vi "Demodlator.vi"(8 "error in (no error)":errorcluster, 10 "Waveform in":waveform(dbl), 11 "ISO 15693 DOWN in":refnum<class "ISO 15693 DOWN.lvclass">) -> (0 "error out":errorcluster, 2 "Waveform out":waveform(dbl), 3 "ISO 15693 DOWN out":refnum<class "ISO 15693 DOWN.lvclass">)   [LabVIEW 2019, in "ISO 15693 DOWN.lvclass"]
uses:
  ISO 15693 DOWN.lvclass
  TypeDef/Store.ctl
  ISO 15693 DOWN.lvclass/ISO 15693 DOWN.ctl
  <vilib>/addons/Modulation/Analog/support/mod_Set Error Source.vi
  <vilib>/addons/Modulation/Analog/MT Downconvert Passband (Real).vi
  <vilib>/addons/Modulation/Analog/MT Demodulate AM (DSB).vi
  <vilib>/addons/Modulation/Digital/Support/Common/Validators/mod_Generate Filter Coefficients Validate.vi
  <vilib>/addons/Modulation/Digital/General/subVIs/mod_Generate Filter Coefficients.vi
  <vilib>/addons/Modulation/Digital/General/MT Generate ASK system parameters (M).vi
  <vilib>/addons/Modulation/niAMT.lvlib
  <vilib>/addons/Modulation/niDMT.lvlib
  RFID system.lvclass
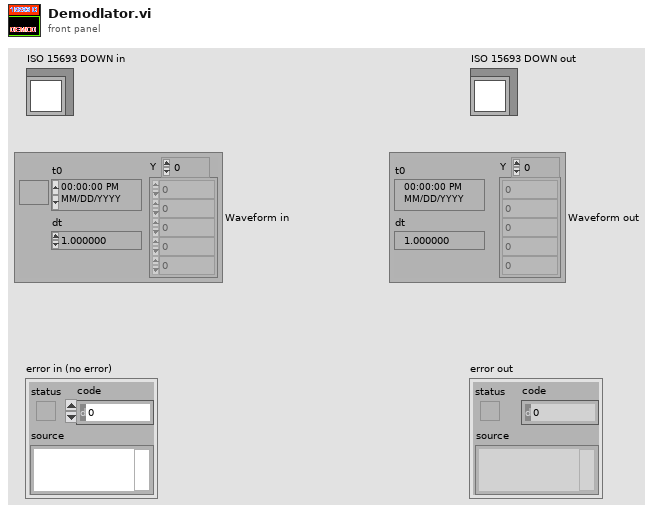
[diagram p1: front panel]
types:
  T1 = typedef "Store.ctl" = enum16{"envelope", "noise", "demSubCar", "CH_frame", "Decode", "demodulate", "in", "out", "sum", "subCarrier", "frame", "command", "encode", "modulate", "encode_UP", "modulate_up", "demod_up", "envelop_up", "sum_up", "out_up", "in_up"}
  T2 = enum16{"none", "Raised Cosine", "Root Raised Cos", "Gaussian"}
  T3 = enum16{"FSK", "PSK", "QAM", "MSK", "PAM", "ASK", "CPM"}
  T4 = cluster{"passband ripple (dB)":dbl, "stopband start (Hz)":dbl, "stopband gain (dB)":dbl, "compute filter stopband ? (T)":bool}
  T5 = typedef "niAMT.lvlib/Complex Data Waveform.ctl" = cluster{"t0":dbl, "dt":dbl, "Y":cdb[]}
  T6 = cluster{"samples per symbol (16)":i32, "symbol map":cdb[]}
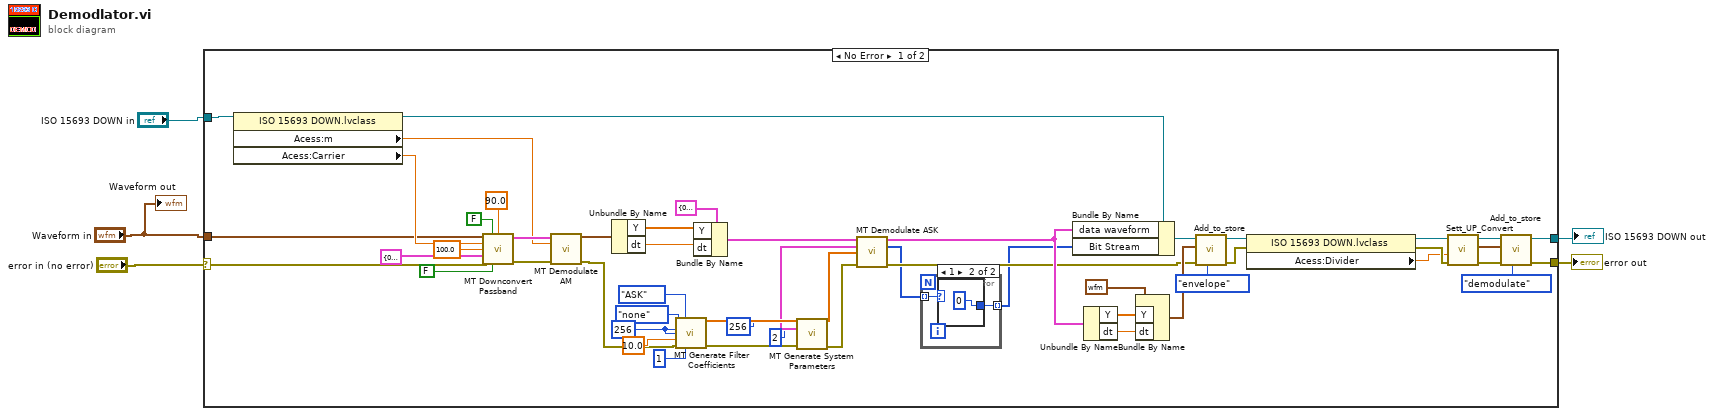
[diagram p0: block diagram]
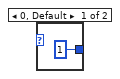
[diagram p2: hidden frame]
diagram:
  n1 = case shown="No Error" "error in (no error)" {
    selector: "error in (no error)" -> [w10 w61]
    tunnel: "ISO 15693 DOWN in" -> [w12 w62]
    tunnel: [w9 w62] -> w2
    tunnel: "Waveform in" -> [w11 _]
    tunnel: [w8 w61] -> w3
    frame No Error {
      w40 = 256 ("pulse shaping samples per symbol (16)")
      n2 = property class="ISO 15693 DOWN.lvclass"(reference=w12) -> (reference out=w32:refnum<class "ISO 15693 DOWN.lvclass">, "Acess:m"=w14:dbl, "Acess:Carrier"=w13:dbl)  [unwired: 1 in, 1 out]
      n3 = call-poly <vilib>:"MT Downconvert Passband.vi"("Waveform"=w11, "reset? (F)"=FALSE, "initial phase (deg)"=90.0, "carrier frequency (Hz)"=w13, "passband bandwidth (Hz)"=100.0, "advanced filter parameters"=T4 {"passband ripple (dB)"=0.01, "stopband start (Hz)"=0.0, "stopband gain (dB)"=-96.0, "compute filter stopband ? (T)"=TRUE}, "error in (no error)"=w10, "enable filter (T)"=FALSE) -> ("downconverted waveform (complex baseband)"=w56:T5, "error out"=w55:errorcluster)  [unwired: 4 in, 2 out]
      n4 = call-poly <vilib>:"MT Demodulate AM.vi"("AM modulated waveform"=w56, "modulation index"=w14, "error in (no error)"=w55) -> ("AM demodulated waveform"=w35:waveform(dbl), "error out"=w34:errorcluster)  [unwired: 10 in, 1 out]
      n5 = Unbundle By Name(w35) -> ("Y"=w47:dbl[], "dt"=w48:dbl)
      n6 = call <vilib>:"MT Generate Filter Coefficients.vi"("pulse shaping filter (none)"=T2."none", "modulation type"=T3."ASK", "pulse shaping samples per symbol (16)"=w40, "matched samples per symbol (16)"=w40, "filter parameter"=10.0, "error in (no error)"=w34, "filter length (symbols)"=1) -> ("pulse shaping filter coefficients"=w46:dbl[], "error out"=w44:errorcluster)  [unwired: 7 out]
      n7 = Bundle By Name(cluster=cluster{"t0":dbl, "dt":dbl, "Y":dbl[]} {"t0"=0.0, "dt"=0.0, "Y"=[]} ("AM modulated waveform"), "Y"=w47, "dt"=w48) -> (w49:cluster{"t0":dbl, "dt":dbl, "Y":dbl[]})
      n8 = call-poly <vilib>:"MT Generate System Parameters.vi"("samples per symbol (16)"=256, "M-ASK (2)"=2, "error in (no error)"=w44) -> ("ASK system parameters"=w45:T6, "error out"=w33:errorcluster)  [unwired: 11 out]
      n9 = call <vilib>:"MT Demodulate ASK.vi"("input complex waveform"=w49, "ASK system parameters"=w45, "matched filter coefficients"=w46, "error in (no error)"=w33) -> ("recovered complex waveform"=w27:T5, "output bit stream"=w7:i8[], "error out"=w25:errorcluster)  [unwired: 7 in, 2 out]
      n10 = for {
        tunnel: w7 -> [w58] mode=indexing
        tunnel: [w57] -> w6 mode=indexing
        n11 = case shown="1" w58 {
          tunnel: [u8 1 ("index") u8 0 ("index")] -> w57
          frame 0, Default {
          }
          frame 1 {
          }
        }
      }
      n12 = Bundle By Name(cluster=w32, "data waveform"=w27, "Bit Stream"=w6) -> (w31:refnum<class "ISO 15693 DOWN.lvclass">)
      n13 = Unbundle By Name(w27) -> ("Y"=w29:cdb[], "dt"=w28:dbl)
      n14 = Bundle By Name(cluster=waveform(cdb) {"t0"=timestamp(0 s since 1904-01-01), "dt"=1.0, "Y"=[]} ("waveform"), "Y"=w29, "dt"=w28) -> (w26:waveform(cdb))
      n15 = call "Add_to_store.vi"("Store"=Store."envelope", "error in (no error)"=w25, "Waveform"=w26, "RFID system in"=w31) -> ("error out"=w17:errorcluster, "RFID system out"=w23:refnum<class "ISO 15693 DOWN.lvclass">)  [unwired: 6 in]
      n16 = property class="ISO 15693 DOWN.lvclass"(reference=w23, error in=w17) -> (reference out=w18:refnum<class "ISO 15693 DOWN.lvclass">, error out=w16:errorcluster, "Acess:Divider"=w15:dbl)
      n17 = call-dynamic "Sett_UP_Convert.vi"("error in (no error)"=w16, "Divider(1)"=w15, "ISO 15693 DOWN in"=w18) -> ("error out"=w21:errorcluster, "Waveform"=w20:waveform(dbl), "ISO 15693 DOWN out"=w22:refnum<class "ISO 15693 DOWN.lvclass">)  [unwired: 6 in]
      n18 = call "Add_to_store.vi"("Store"=Store."demodulate", "error in (no error)"=w21, "Waveform"=w20, "RFID system in"=w22) -> ("error out"=w8:errorcluster, "RFID system out"=w9:refnum<class "ISO 15693 DOWN.lvclass">)  [unwired: 6 in]
    }
    frame Error {
    }
  }
  "error out" <- w3
  "ISO 15693 DOWN out" <- w2
  "Waveform out" <- "Waveform in"
